vi "SELECT_OUTPUT_CHANNEL.vi"(2 "Channel ID IN":i32=-999999, 3 "DAQmx Global Channel IN":refnum<k21>) -> (0 "DAQmx Global Channel OUT":refnum<k21>, 1 "Channel ID OUT":i32)   [LabVIEW 2013]
doc: "Selects a DAQmx Global Channel given a numeric index, or vice versa."
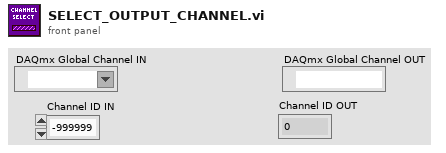
[diagram p1: front panel]
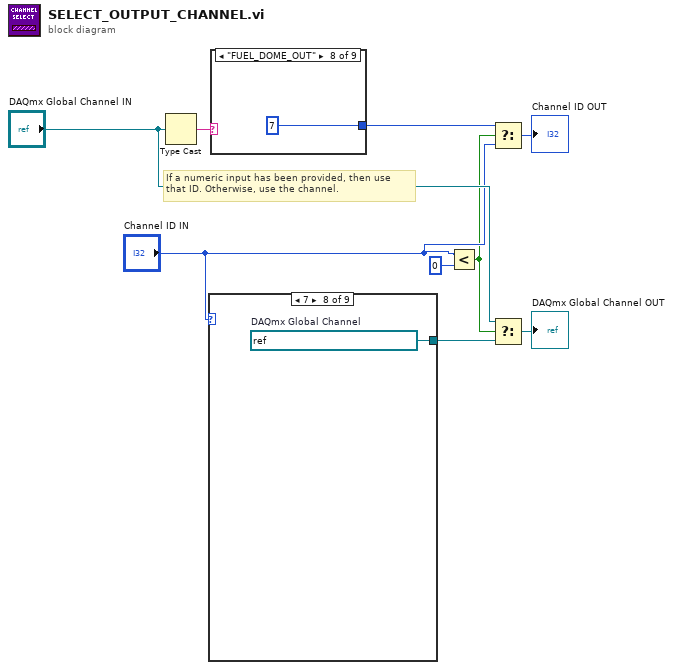
[diagram p0: block diagram]
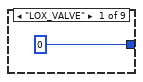
[diagram p2: hidden frame]
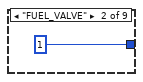
[diagram p3: hidden frame]
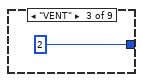
[diagram p4: hidden frame]
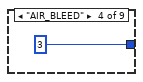
[diagram p5: hidden frame]
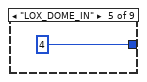
[diagram p6: hidden frame]
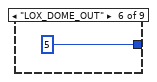
[diagram p7: hidden frame]
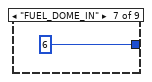
[diagram p8: hidden frame]
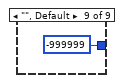
[diagram p9: hidden frame]
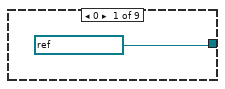
[diagram p10: hidden frame]
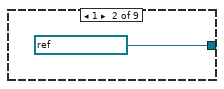
[diagram p11: hidden frame]
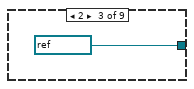
[diagram p12: hidden frame]
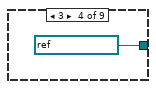
[diagram p13: hidden frame]
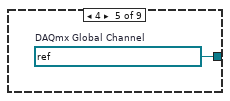
[diagram p14: hidden frame]
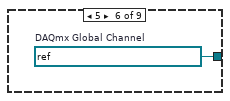
[diagram p15: hidden frame]
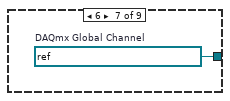
[diagram p16: hidden frame]
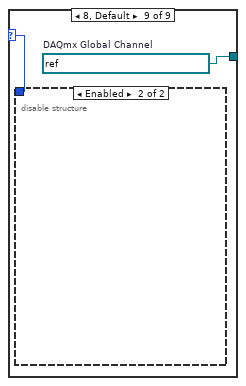
[diagram p17: hidden frame]
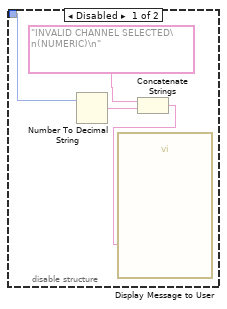
[diagram p18: hidden frame]
diagram:
  # "If a numeric input has been provided, then use \nthat ID. Otherwise, use the channel."
  n1 = Type Cast(x="DAQmx Global Channel IN") -> (*(type *) &x=w6:string)  [unwired: 1 in]
  n2 = case shown="7" "Channel ID IN" {
    selector: "Channel ID IN" -> [_ _ _ _ _ _ _ _ w18]
    tunnel: [refnum<k21> "LOX_VALVE" ("DAQmx Global Channel 2") refnum<k21> "FUEL_VALVE" ("DAQmx Global Channel 2") refnum<k21> "VENT" ("DAQmx Global Channel 2") refnum<k21> "AIR_BLEED" ("DAQmx Global Channel 2") w14 w15 w16 w17 w19] -> w9
    frame 0 {
    }
    frame 1 {
    }
    frame 2 {
    }
    frame 3 {
    }
    frame 4 {
      w14 = refnum<k21> "LOX_DOME_IN"  # DAQmx Global Channel
    }
    frame 5 {
      w15 = refnum<k21> "LOX_DOME_OUT"  # DAQmx Global Channel
    }
    frame 6 {
      w16 = refnum<k21> "FUEL_DOME_IN"  # DAQmx Global Channel
    }
    frame 7 {
      w17 = refnum<k21> "FUEL_DOME_OUT"  # DAQmx Global Channel
    }
    frame 8, Default {
      w19 = refnum<k21> "AIR_BLEED"  # DAQmx Global Channel
      n3 = disable-structure shown="Enabled" {
        disable-tunnel: w18 -> [w23 _]
        frame Disabled {
          n4 = Number To Decimal String(number=w23) -> (decimal integer string=w22:string)  [unwired: 1 in]
          n5 = Concatenate Strings("INVALID CHANNEL SELECTED\n(NUMERIC)\n", w22) -> (w20:string)
          n6 = call "Display Message to User"("Message"=w20) -> ()  [unwired: 9 in, 2 out]
        }
        frame Enabled {
        }
      }
    }
  }
  n7 = case shown="\"FUEL_DOME_OUT\"" w6 {
    tunnel: [0 1 2 3 4 5 6 7 -999999] -> w4
    frame "LOX_VALVE" {
    }
    frame "FUEL_VALVE" {
    }
    frame "VENT" {
    }
    frame "AIR_BLEED" {
    }
    frame "LOX_DOME_IN" {
    }
    frame "LOX_DOME_OUT" {
    }
    frame "FUEL_DOME_IN" {
    }
    frame "FUEL_DOME_OUT" {
    }
    frame "", Default {
    }
  }
  n8 = Less?(x="Channel ID IN", y=0) -> (x < y?=w1:bool)
  n9 = Select(t=w4, s=w1, f="Channel ID IN") -> (s? t:f=→"Channel ID OUT":i32)
  n10 = Select(t="DAQmx Global Channel IN", s=w1, f=w9) -> (s? t:f=→"DAQmx Global Channel OUT":refnum<k21>)
